vi "Send Message to Local Process.vi"(0 "process name":string, 5 "message":T1, 9 "timeout (-1 ms)":i32=-1, 11 "error in":errorcluster) -> (10 "timed out?":bool, 15 "error out":errorcluster)   [LabVIEW 2015, in "TLB` Template.lvlib" / "AMC.lvlib"]
doc: "TLB Prime - Application Template 1.3.0.24\nNorm Kirchner, NI Systems Engineering - NI\nCopyright (c) 2014, NI"
uses:
  AMC.lvlib
  Message.ctl
  Tools/Keyed Array/KeyedArray.ctl
  Tools/Keyed Array/Tools_KeyedArray.lvlib
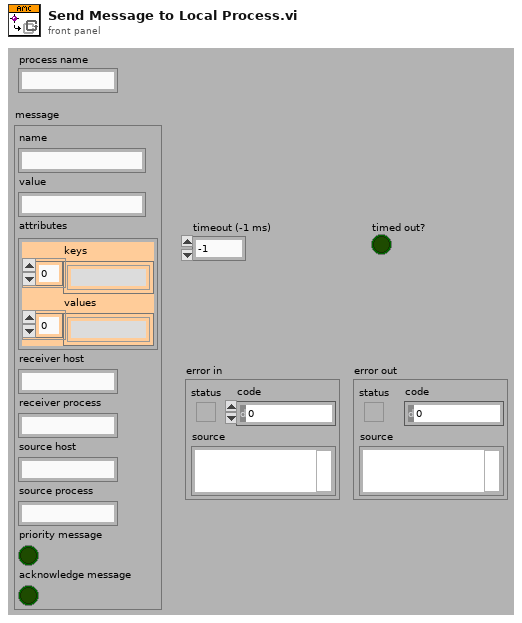
[diagram p1: front panel]
types:
  T1 = typedef "TLB` Template.lvlib/AMC.lvlib/Message.ctl" = cluster{"name":string, "value":string, "attributes":T2, "receiver host":string, "receiver process":string, "source host":string, "source process":string, "priority message":bool, "acknowledge message":bool}
  T2 = typedef "TLB` Template.lvlib/Tools_KeyedArray.lvlib/KeyedArray.ctl" = cluster{"keys":string[], "values":string[]}
  T3 = typedef "TLB` Template.lvlib/AMC.lvlib/Message Queue.ctl" = refnum<queue>
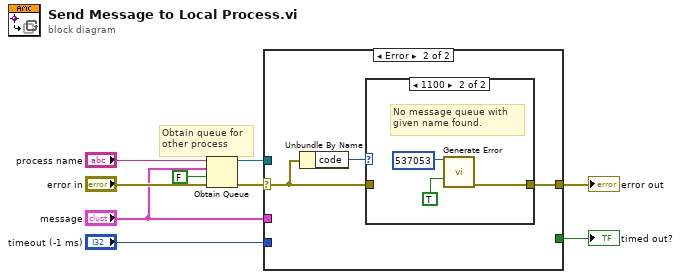
[diagram p0: block diagram]
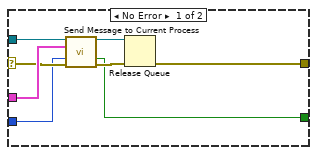
[diagram p2: hidden frame]
diagram:
  # "Obtain queue for\nother process"
  n1 = Obtain Queue(name (unnamed)="process name", element data type="message", create if not found? (T)=FALSE, error in (no error)="error in") -> (queue out=w9:refnum<queue>, error out=w3:errorcluster)  [unwired: 1 in, 1 out]
  n2 = case shown="Error" w3 {
    selector: w3 -> [w13 w18]
    tunnel: w9 -> [w16 _]
    tunnel: [w17 w19] -> w7
    tunnel: "message" -> [w15 _]
    tunnel: "timeout (-1 ms)" -> [w11 _]
    tunnel: [w10 _] -> w1
    frame No Error {
      n3 = call "Send Message to Current Process.vi"("message queue in"=w16, "message"=w15, "timeout (-1 ms)"=w11, "error in"=w13) -> ("message queue out"=w14:T3, "timed out?"=w10:bool, "error out"=w12:errorcluster)  [unwired: 9 in]
      n4 = Release Queue(queue=w14, error in (no error)=w12) -> (error out=w17:errorcluster)  [unwired: 3 out]
    }
    frame Error {
      n5 = Unbundle By Name(w18) -> ("code"=w20:i32)
      n6 = case shown="1100" w20 {
        tunnel: [w21 w22] -> w19
        tunnel: w18 -> [w21 _]
        frame 0, Default {
        }
        frame 1100 {
          # "No message queue with given name found."
          n7 = call "Generate Error.vi"("code"=537053, "status (F)"=TRUE) -> ("error out"=w22:errorcluster)  [unwired: 13 in]
        }
      }
    }
  }
  "error out" <- w7
  "timed out?" <- w1
